vi "SSC DCPower Send Software Edge Trigger.vi"(0 "DCPower SSC in":T2[](array[typedef]), 5 "Trigger to Send":T1=1036 caption="signal" items=["Start Trigger"=1034, "Source Trigger"=1035, "Measure Trigger"=1036, "Sequence Advance Trigger"=1037, "Pulse Trigger"=1053], 11 "error in":errorcluster) -> (4 "DCPower SSC out":T2[](array[typedef]), 15 "error out":errorcluster)   [LabVIEW 2020]
doc: "This VI sends a software edge trigger to every session"
uses:
  SSC DCPower.ctl
  <instrlib>/niDCPower/nidcpower.llb/niDCPower Send Software Edge Trigger - Signal.ctl
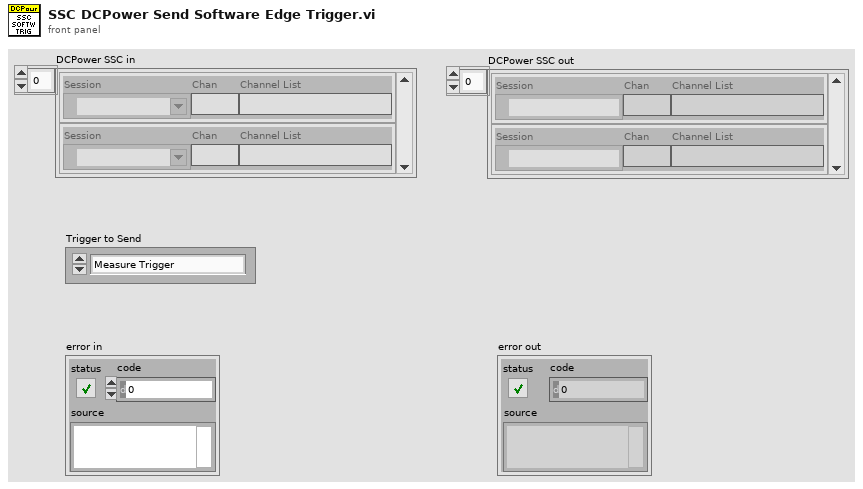
[diagram p1: front panel]
types:
  T1 = typedef "niDCPower Send Software Edge Trigger - Signal.ctl" = i32
  T2 = typedef "SSC DCPower.ctl" = cluster{"Session":refnum<k15>, "Chan":string, "Channel List":string}
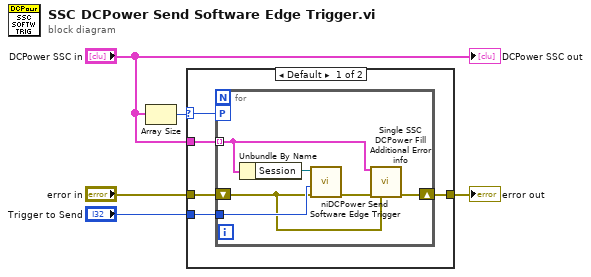
[diagram p0: block diagram]
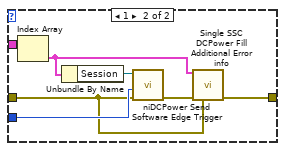
[diagram p2: hidden frame]
diagram:
  n1 = Array Size(array="DCPower SSC in") -> (size(s)=w2:i32)
  n2 = case shown="Default" w2 {
    selector: w2 -> [w7 _]
    tunnel: [w10 w23] -> w5
    tunnel: "Trigger to Send" -> [w9 w22]
    tunnel: "error in" -> [w8 w21]
    tunnel: "DCPower SSC in" -> [w6 w20]
    frame Default {
      n3 = for {
        tunnel: w6 -> [w12] mode=indexing
        tunnel: w9 -> [w15]
        workers-P: w7 -> [_]
        shift-right: [w13] -> w10
        shift-left: w8 -> [w11]
        n4 = Unbundle By Name(w12) -> ("Session"=w14:refnum<k15>)
        n5 = call <instrlib>:"niDCPower Send Software Edge Trigger.vi"("error in (no error)"=w11, "signal"=w15, "instrument handle"=w14) -> ("error out"=w16:errorcluster)  [unwired: 7 in, 1 out]
        n6 = call "Single SSC DCPower Fill Additional Error info.vi"("DCPower SSC in"=w12, "error in"=w16, "previous error in"=w11) -> ("error out"=w13:errorcluster)  [unwired: 12 in]
      }
    }
    frame 1 {
      n7 = Index Array(array=w20) -> (element=w17:T2)  [unwired: 1 in]
      n8 = Unbundle By Name(w17) -> ("Session"=w18:refnum<k15>)
      n9 = call <instrlib>:"niDCPower Send Software Edge Trigger.vi"("error in (no error)"=w21, "signal"=w22, "instrument handle"=w18) -> ("error out"=w19:errorcluster)  [unwired: 7 in, 1 out]
      n10 = call "Single SSC DCPower Fill Additional Error info.vi"("DCPower SSC in"=w17, "error in"=w19, "previous error in"=w21) -> ("error out"=w23:errorcluster)  [unwired: 12 in]
    }
  }
  "error out" <- w5
  "DCPower SSC out" <- "DCPower SSC in"
